vi "Comm Serial Read All Bytes.vi"(8 "error in (no error)":errorcluster, 11 "niDTS Comm Serial in":refnum<class "niDTS Comm Serial.lvclass">) -> (0 "error out":errorcluster, 2 "Read":string, 3 "niDTS Comm Serial out":refnum<class "niDTS Comm Serial.lvclass">)   [LabVIEW 2015, in "niDTS CommLib.lvlib" / "niDTS Comm Serial.lvclass"]
uses:
  niDTS Comm Serial.lvclass
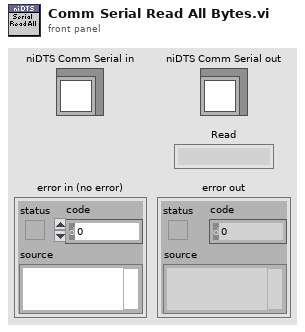
[diagram p1: front panel]
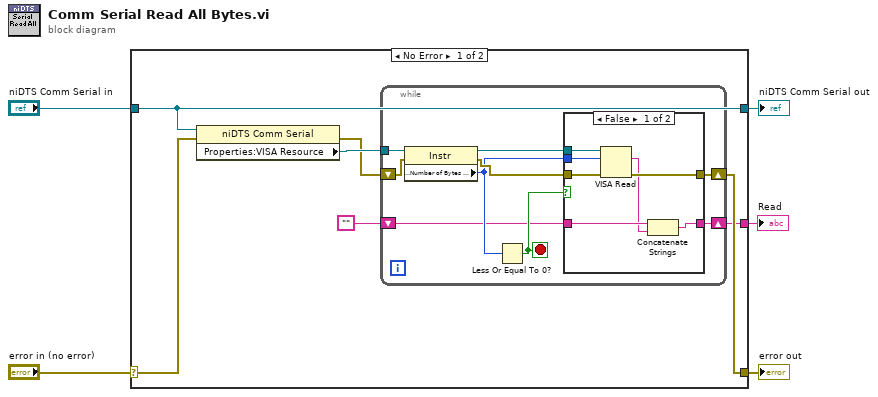
[diagram p0: block diagram]
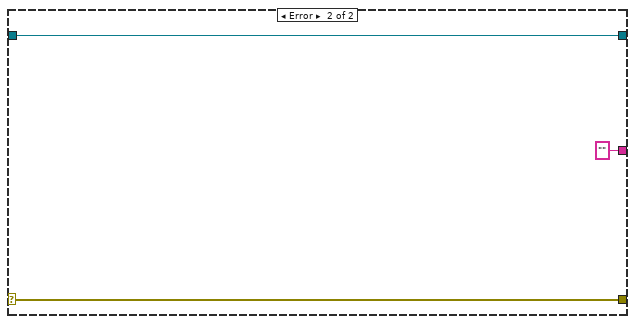
[diagram p3: hidden frame]
diagram:
  n1 = case shown="No Error" "error in (no error)" {
    selector: "error in (no error)" -> [w11 w33]
    tunnel: [w7 w33] -> w4
    tunnel: [w12 w32] -> w2
    tunnel: "niDTS Comm Serial in" -> [w12 w32]
    tunnel: [w6 ""] -> w1
    frame No Error {
      n2 = property class="niDTS Comm Serial"(reference=w12, error in=w11) -> (error out=w9:errorcluster, "Properties:VISA Resource"=w10:refnum<visa-resource-name>)  [unwired: 1 out]
      n3 = while {
        tunnel: w10 -> [w19]
        shift-right: [w16] -> w7
        shift-left: w9 -> [w15]
        shift-right: [w13] -> w6
        shift-left: "" -> [w14]
        stop <- w17 stop-if-true
        n4 = property class="Instr"(reference=w19, error in=w15) -> (reference out=w20:refnum<visa-resource-name>, error out=w21:errorcluster, "Serial Settings:Number of Bytes at Serial Port"=w18:u32)
        n5 = Less Or Equal To 0?(x=w18) -> (x <= 0?=w17:bool)
        n6 = case shown="False" w17 {
          tunnel: w21 -> [w28 w29]
          tunnel: w20 -> [w27 _]
          tunnel: w18 -> [w26 _]
          tunnel: [w25 w29] -> w16
          tunnel: w14 -> [w23 w30]
          tunnel: [w24 w30] -> w13
          frame False {
            n7 = VISA Read(VISA resource name=w27, byte count=w26, error in (no error)=w28) -> (read buffer=w22:string, error out=w25:errorcluster)  [unwired: 2 out]
            n8 = Concatenate Strings(w23, w22) -> (w24:string)
          }
          frame True {
          }
        }
      }
    }
    frame Error {
    }
  }
  "error out" <- w4
  "niDTS Comm Serial out" <- w2
  "Read" <- w1
